vi "DIM-Error.vi"() -> (2 "DIM Error":bool)   [LabVIEW 2014, in "Panels.lvlib"]
uses:
  Panels.lvlib
  Instance           1 17Saved   DIM-Error .vi
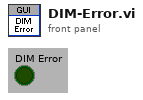
[diagram p1: front panel]
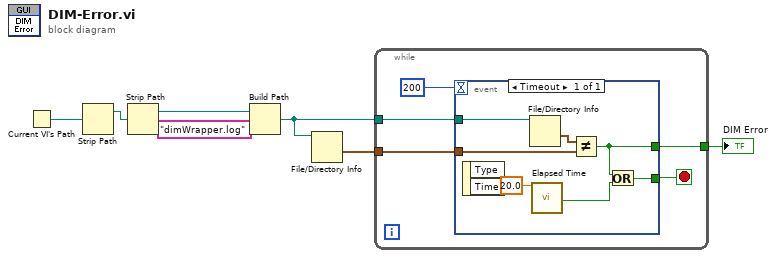
[diagram p0: block diagram]
diagram:
  n1 = Current VI's Path() -> (path=w1:path)
  n2 = Strip Path(path=w1) -> (stripped path=w2:path)  [unwired: 1 out]
  n3 = Strip Path(path=w2) -> (stripped path=w6:path)  [unwired: 1 out]
  n4 = Build Path(base path=w6, name or relative path="dimWrapper.log") -> (appended path=w4:path)
  n5 = File/Directory Info(path=w4) -> (last mod=w5:timestamp)  [unwired: 1 in, 6 out]
  n6 = while {
    tunnel: w5 -> [w11]
    tunnel: w4 -> [w10]
    tunnel: [w8] -> w3
    stop <- w9 stop-if-true
    n7 = event shown="[0] Timeout" {
      selector: _ -> [_]
      dyn-events: _ -> [_]
      timeout: 200 -> [_]
      tunnel: w11 -> [w17]
      tunnel: w10 -> [w19]
      tunnel: [w16] -> w9
      tunnel: [w15] -> w8
      event Timeout {
        n8 = event-data() -> ()  [unwired: 1 in, 2 out]
        n9 = File/Directory Info(path=w19) -> (last mod=w18:timestamp)  [unwired: 1 in, 6 out]
        n10 = call "Elapsed Time"("Time Target (s)"=20.0) -> ("Time has Elapsed"=w13:bool)  [unwired: 11 in, 7 out]
        n11 = Not Equal?(x=w18, y=w17) -> (x != y?=w15:bool)
        n12 = Or(x=w15, y=w13) -> (x .or. y?=w16:bool)
      }
    }
  }
  "DIM Error" <- w3
